vi "FRA example-AndreTec.vi"() -> ()   [LabVIEW 2014]
doc: "André Romero - 2016\nandretec@ifsc.usp.br\nIFSC - USP"
uses:
  <vilib>/Analysis/Matrix/Datatypes/RealMatrix.ctl
  C:/UserLabs/Andre/Nova-Autolab/Labview/Autolab SDK 1.11/EcoChemie.Autolab.Sdk.dll
  EcoChemie.Autolab.Sdk.dll
  <vilib>/Instr/_visa.llb/VISA Configure Serial Port (Instr).vi
  <vilib>/Utility/file.llb/Write To Spreadsheet File (DBL).vi
  <vilib>/Analysis/Matrix/NI_Matrix.lvlib
panel:
  in  "String":string="Wait !!!! Instrument is initializing ...."
  in  "Start Measurement":bool
  out "Sensor":i32=1
  out "error out":errorcluster={"status"=TRUE, "code"=-1073807343, "source"="Property Node (arg 1) in VISA Configure Serial Port (Instr).vi->Measuring Complete - AndreTec-2.vi"}
  out "VISA resource name out":refnum<visa-resource-name>="COM3"
  in  "N. Sensors":i32=3 min=1 max=8
  out "Measurement":cluster{dbl[], dbl[]}(graph)
  out "Points":i32=478
  in  "Abort":bool
  in  "Y axis Signal":string(combo)="WE(1).Current"
  in  "X axis Signal":string(combo)="WE(1).Potential"
  out "Measured data":cluster{"Y":dbl[], "Y":dbl[]}[](graph)
  out "X axis value":dbl=-1.1810302734375e-08
  out "Y axis value":dbl=3.0517578124972244e-06
  out "Measurement active":bool
  out "Blacklisted Commands detected":bool
  in  "Load Procedure (.nox)":path=path "C:/Users/user/Documents/My Procedures 1.11/Procedures/FRA impedance potentiostatic.nox"
  out "Autolab Connected":bool
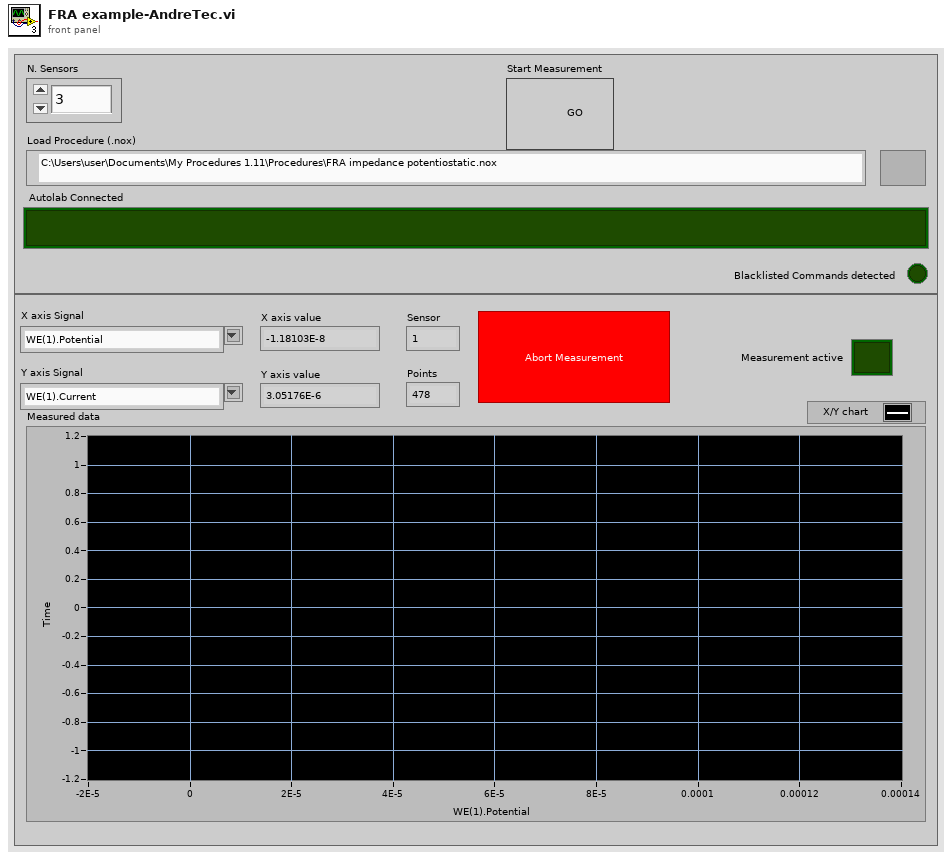
[diagram p1: front panel]
types:
  T1 = typedef "NI_Matrix.lvlib/RealMatrix.ctl" = dbl[][]
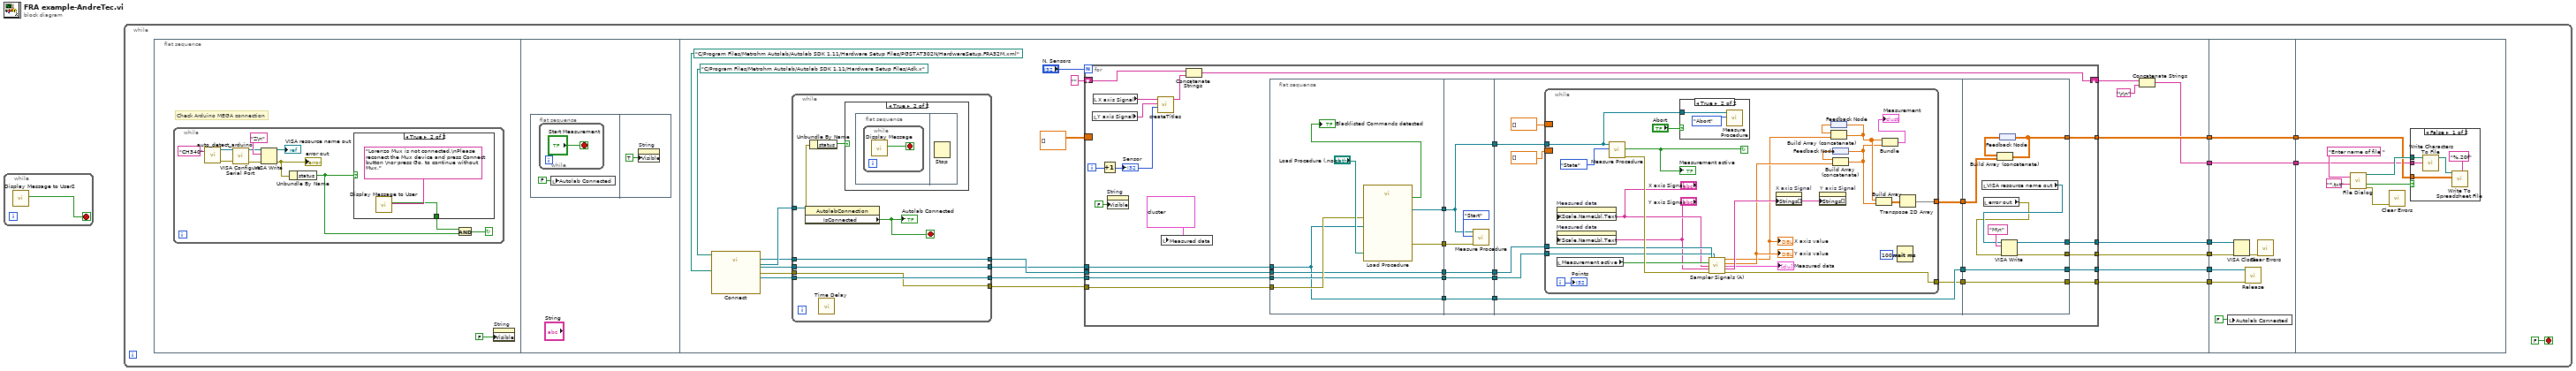
[diagram p0: block diagram]
diagram:
  n1 = while {
    stop <- w1 stop-if-true
    n2 = call "Display Message to User2"() -> ("OK"=w1:bool)  [unwired: 10 in, 1 out]
  }
  n3 = while {
    stop <- FALSE stop-if-true
    n4 = flat-sequence {
      tunnel: [w36] -> w9
      tunnel: [w34] -> w7
      tunnel: [w32] -> w5
      tunnel: [w31] -> w4
      tunnel: [w30] -> w3
      tunnel: [w29] -> w2
      tunnel: w9 -> [w154]
      tunnel: [w154] -> w8
      tunnel: w7 -> [w153]
      tunnel: [w153] -> w6
      tunnel: w5 -> [w150]
      tunnel: w4 -> [w149]
      tunnel: w3 -> [w148]
      tunnel: w2 -> [w147]
      tunnel: w8 -> [w158]
      tunnel: w6 -> [w157]
      frame #0 {
        # "Check Arduino MEGA connection"
        n5 = while {
          stop <- w14 continue-if-true
          n6 = call "auto_detect_arduino.vi"("instr name"="CH340") -> ("VISA resource name"=w22:refnum<visa-resource-name>, "error out"=w15:errorcluster)  [unwired: 1 in, 1 out]
          n7 = call-poly "VISA Configure Serial Port"("VISA resource name"=w22, "error in (no error)"=w15) -> ("VISA resource name out"=w19:refnum<visa-resource-name>, "error out"=w18:errorcluster)  [unwired: 7 in, 5 out]
          n8 = VISA Write(VISA resource name=w19, write buffer="Z\n" ("Command"), error in (no error)=w18) -> (VISA resource name out=→"VISA resource name out":refnum<visa-resource-name>, error out=w16:errorcluster)  [unwired: 1 out]
          "error out" <- w16
          n9 = Unbundle By Name(w16) -> ("status"=w13:bool)
          n10 = case shown="True" w13 {
            tunnel: [_ w23] -> w12
            frame False {
            }
            frame True {
              n11 = call "Display Message to User"("Message"="Lorenzo Mux is not connected.\nPlease reconect the Mux device and press Connect button \nor press Go, to continue without Mux.") -> ("Connect"=w23:bool)  [unwired: 9 in, 1 out]
            }
          }
          n12 = And(x=w12, y=w13) -> (x .and. y?=w14:bool)
        }
        n13 = property on="String" class="Str"("Visible"=FALSE) -> ()  [unwired: 2 in, 2 out]
      }
      frame #1 {
        n14 = flat-sequence {
          frame #0 {
            n15 = while {
              stop <- "Start Measurement" stop-if-true
            }
            n16 = local write "Autolab Connected"(FALSE ("Autolab Connected")) -> ()
          }
          frame #1 {
            n17 = property on="String" class="Str"("Visible"=TRUE) -> ()  [unwired: 2 in, 2 out]
          }
        }
      }
      frame #2 {
        n18 = call "Connect.vi"("Embedded Exe File"=path "C:/Program Files/Metrohm Autolab/Autolab SDK 1.11/Hardware Setup Files/Adk.x", "Hardware Setup File"=path "C:/Program Files/Metrohm Autolab/Autolab SDK 1.11/Hardware Setup Files/PGSTAT302N/HardwareSetup.FRA32M.xml") -> ("Sampler"=w46:refnum<k24>, "AutolabConnection"=w47:refnum<k24>, "instrument"=w44:refnum<k24>, "Ei"=w40:refnum<k24>, "error out"=w42:errorcluster)  [unwired: 1 in, 8 out]
        n19 = while {
          tunnel: w47 -> [w144]
          tunnel: w46 -> [w141]
          tunnel: [w141] -> w45
          tunnel: w44 -> [w140]
          tunnel: [w140] -> w43
          tunnel: w40 -> [w139]
          tunnel: [w139] -> w28
          tunnel: w42 -> [w138]
          tunnel: [w138] -> w41
          stop <- w145 stop-if-true
          n20 = property class="AutolabConnection"(reference=w144) -> (error out=w142:errorcluster, "IsConnected"=w145:bool)  [unwired: 1 in, 1 out]
          "Autolab Connected" <- w145
          n21 = Unbundle By Name(w142) -> ("status"=w143:bool)
          n22 = call "Time Delay"() -> ()  [unwired: 2 in, 10 out]
          n23 = case shown="True" w143 {
            frame False {
            }
            frame True {
              n24 = flat-sequence {
                frame #0 {
                  n25 = while {
                    stop <- w146 stop-if-true
                    n26 = call "Display Message"() -> ("OK"=w146:bool)  [unwired: 10 in, 1 out]
                  }
                }
                frame #1 {
                  n27 = Stop() -> ()  [unwired: 1 in]
                }
              }
            }
          }
        }
        n28 = for {
          N: "N. Sensors" -> [_]
          tunnel: [w68] -> w32
          tunnel: [w67] -> w31
          tunnel: [w66] -> w30
          tunnel: [w65] -> w29
          tunnel: w41 -> [w64]
          tunnel: w43 -> [w63]
          tunnel: w45 -> [w62]
          tunnel: w28 -> [w61]
          tunnel: [w58] -> w36
          border: T1 [] ("Real Matrix") -> [_]
          shift-right: [w51] -> w35
          shift-left: "" -> [w53]
          i -> [w57]
          n29 = local read "Y axis Signal"() -> (w54:string)
          n30 = local read "X axis Signal"() -> (w55:string)
          n31 = Increment(x=w57) -> (x+1=w50:i32)
          "Sensor" <- w50
          n32 = property on="String" class="Str"("Visible"=FALSE) -> ()  [unwired: 2 in, 2 out]
          n33 = call "createTitles.vi"("Numeric"=w50, "Y axis Signal"=w54, "X axis Signal"=w55) -> ("String"=w52:string)  [unwired: 8 in]
          n34 = local write "Measured data"(cluster{"Y":dbl[], "Y":dbl[]}[] [{"Y"=array[2393 elements], "Y"=array[2393 elements]}] ("Measured data")) -> ()
          n35 = Concatenate Strings(w53, w52) -> (w51:string)
          n36 = flat-sequence {
            tunnel: [w85] -> w79
            tunnel: [w84] -> w78
            tunnel: [w82] -> w77
            tunnel: [w81] -> w76
            tunnel: [w80] -> w75
            tunnel: w63 -> [w80]
            tunnel: w64 -> [w83]
            tunnel: w62 -> [w82]
            tunnel: w61 -> [w81]
            tunnel: w79 -> [w91]
            tunnel: w78 -> [w92]
            tunnel: [w91] -> w74
            tunnel: w77 -> [w90]
            tunnel: w76 -> [w89]
            tunnel: [w90] -> w73
            tunnel: [w89] -> w72
            tunnel: [w88] -> w71
            tunnel: w75 -> [w88]
            tunnel: w74 -> [w101]
            tunnel: w73 -> [w100]
            tunnel: w72 -> [w99]
            tunnel: w71 -> [w98]
            tunnel: [w98] -> w70
            tunnel: [w94] -> w69
            tunnel: [w97] -> w59
            tunnel: w70 -> [w137]
            tunnel: w69 -> [w136]
            tunnel: [w137] -> w68
            tunnel: [w136] -> w67
            tunnel: [w132] -> w66
            tunnel: [w131] -> w65
            tunnel: w59 -> [w130]
            tunnel: [w128] -> w58
            frame #0 {
              n37 = call "Load Procedure.vi"("error in (no error)"=w83, "Procedure"="Load Procedure (.nox)", "Instrument"=w80) -> ("error out"=w84:errorcluster, "Contains"=→"Blacklisted Commands detected":bool, "LoadProcedure"=w85:refnum<k24>)  [unwired: 6 out]
            }
            frame #1 {
              n38 = call "Measure Procedure.vi"("error in"=w92, "Request for procedure"=enum16{"State", "Save", "Abort", "Start"}."Start", "LoadProcedure"=w91) -> ()  [unwired: 1 in, 8 out]
            }
            frame #2 {
              n39 = while {
                tunnel: w101 -> [w119]
                tunnel: w100 -> [w120]
                tunnel: w99 -> [w104]
                tunnel: [w107] -> w97
                border: dbl[] [] -> [_]
                border: dbl[] [] -> [_]
                tunnel: [w106] -> w94
                i -> [w116]
                stop <- w111 continue-if-true
                n40 = property on="Measured data" class="XYGraph (strict)"("XScale.NameLbl.Text"="X axis Signal") -> ()  [unwired: 2 in, 2 out]
                n41 = property on="Measured data" class="XYGraph (strict)"("YScale.NameLbl.Text"="Y axis Signal") -> ()  [unwired: 2 in, 2 out]
                n42 = local read "Measurement active"() -> (w122:bool)
                n43 = call "Measure Procedure.vi"("Request for procedure"=enum16{"State", "Save", "Abort", "Start"}."State", "LoadProcedure"=w119) -> ("error out"=w123:errorcluster, "IsMeasuring"=w111:bool)  [unwired: 2 in, 6 out]
                "Measurement active" <- w111
                n44 = case shown="True" "Abort" {
                  tunnel: w119 -> [_ w126]
                  frame False {
                  }
                  frame True {
                    n45 = call "Measure Procedure.vi"("Request for procedure"=enum16{"State", "Save", "Abort", "Start"}."Abort", "LoadProcedure"=w126) -> ()  [unwired: 2 in, 8 out]
                  }
                }
                n46 = call "Sampler Signals (A).vi"("IsMeasuring"=w122, "EI"=w104, "Sampler"=w120, "Signal X"="X axis Signal", "Signal Y"="Y axis Signal", "error in"=w123) -> ("X"=w105:dbl, "Y"=w113:dbl, "XY Graph"=→"Measured data":cluster{"Y":dbl[], "Y":dbl[]}[], "GetSignals"=w125:string[], "error out"=w106:errorcluster)  [unwired: 4 in, 1 out]
                "Y axis value" <- w113
                "X axis value" <- w105
                n47 = property on="X axis Signal" class="CmbBox"("Strings[]"=w125) -> ()  [unwired: 2 in, 2 out]
                n48 = property on="Y axis Signal" class="CmbBox"("Strings[]"=w125) -> ()  [unwired: 2 in, 2 out]
                n49 = feedback #1() -> (w115:dbl[])
                n50 = Build Array (concatenate)(w115, w105) -> (w109:dbl[])
                n51 = feedback-in #1(w109) -> ()
                n52 = feedback #2() -> (w114:dbl[])
                n53 = Build Array (concatenate)(w114, w113) -> (w108:dbl[])
                n54 = feedback-in #2(w108) -> ()
                n55 = Build Array(w109, w108) -> (w110:dbl[][])
                n56 = Bundle(w109, w108) -> (→"Measurement":cluster{dbl[], dbl[]})  [unwired: 1 in]
                n57 = Wait (ms)(milliseconds to wait=u32 100) -> ()  [unwired: 1 out]
                n58 = Transpose 2D Array(2D array=w110) -> (transposed array=w107:dbl[][])
                "Points" <- w116
              }
            }
            frame #3 {
              n59 = local read "VISA resource name out"() -> (w134:refnum<visa-resource-name>)
              n60 = local read "error out"() -> (w133:errorcluster)
              n61 = feedback #3() -> (w129:T1)
              n62 = Build Array (concatenate)(w129, w130) -> (w128:T1)
              n63 = feedback-in #3(w128) -> ()
              n64 = VISA Write(VISA resource name=w134, write buffer="M\n" ("Command"), error in (no error)=w133) -> (VISA resource name out=w132:refnum<visa-resource-name>, error out=w131:errorcluster)  [unwired: 1 out]
            }
          }
        }
        n65 = Concatenate Strings(w35, "\r\n") -> (w34:string)
      }
      frame #3 {
        n66 = local write "Autolab Connected"(FALSE ("Autolab Connected")) -> ()
        n67 = VISA Close(VISA resource name=w148, error in (no error)=w147) -> (error out=w151:errorcluster)
        n68 = call "Release.vi"("error in (no error)"=w149, "Instrument"=w150) -> ()  [unwired: 1 in, 9 out]
        n69 = call <vilib>:"Clear Errors.vi"("error in (no error)"=w151) -> ()  [unwired: 5 in, 2 out]
      }
      frame #4 {
        n70 = call "File Dialog"("prompt"="Enter name of file ", "pattern (all files)"="*.txt") -> ("selected path"=w159:path, "cancelled"=w155:bool, "error out"=w156:errorcluster)  [unwired: 10 in, 1 out]
        n71 = call <vilib>:"Clear Errors.vi"("error in (no error)"=w156) -> ()  [unwired: 5 in, 2 out]
        n72 = case shown="False" w155 {
          tunnel: w159 -> [w166 _]
          tunnel: w158 -> [w163 _]
          tunnel: w157 -> [w162 _]
          frame False {
            n73 = call <vilib>:"Write Characters To File.vi"("character string"=w162, "file path (dialog if empty)"=w166) -> ("new file path (Not A Path if cancelled)"=w165:path)  [unwired: 3 in]
            n74 = call-poly <vilib>:"Write To Spreadsheet File.vi"("format (%.3f)"="%.20f", "2D data"=w163, "file path (dialog if empty)"=w165) -> ()  [unwired: 5 in, 1 out]
          }
          frame True {
          }
        }
      }
    }
  }
